vi "LabVIEW1.vi"() -> ()   [LabVIEW 2023]
panel:
  out "Class Average Score":dbl
  out "Number of Students":i32
  in  "Table Control":string[][](table)
  # "INPUT"
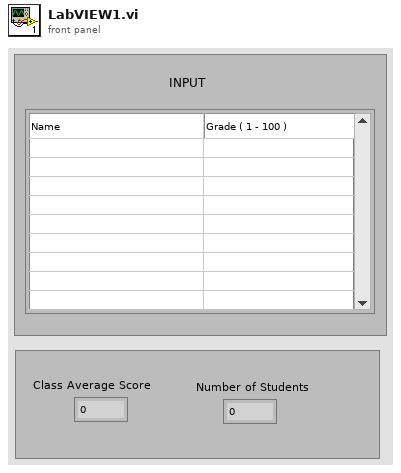
[diagram p1: front panel]
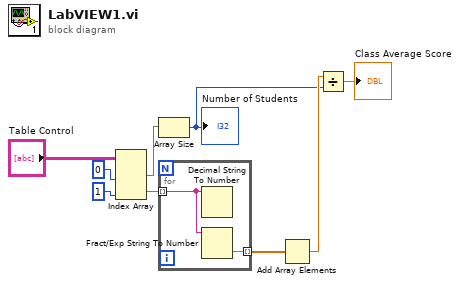
[diagram p0: block diagram]
diagram:
  n1 = Index Array(array="Table Control", index (col) #1=0 ("disabled index (col)"), index (col) #2=1 ("index (col)")) -> (element #1=w6:string[], element #2=w5:string[])  [unwired: 2 in]
  n2 = Array Size(array=w6) -> (size(s)=w2:i32)
  "Number of Students" <- w2
  n3 = for {
    tunnel: w5 -> [w11] mode=indexing
    tunnel: [w10] -> w4 mode=indexing
    n4 = Decimal String To Number(string=w11) -> ()  [unwired: 2 in, 2 out]
    n5 = Fract/Exp String To Number(string=w11) -> (number=w10:dbl)  [unwired: 3 in, 1 out]
  }
  n6 = Add Array Elements(numeric array=w4) -> (sum=w3:dbl)
  n7 = Divide(x=w3, y=w2) -> (x/y=→"Class Average Score":dbl)
